vi "io.interface.vi"(7 "Caller":string, 8 "error in":errorcluster, 9 "record filename.* (disabled if empty)":string, 10 "IO Value":variant, 11 "IO Name in":string) -> (0 "error out":errorcluster, 1 "unCalibrated":u16, 2 "Value out":dbl, 3 "IoConf out":T1={"ADDR"=0, "Label"="", "Type"=enum."DI", "Mode"=enum."RIO", "Value"="", "Tags"="", "calibration"=[]} {"calibration"."Y" format="%#.3f"; "calibration"."X" format="%#.3f"; "ADDR" format="%04d"}, 4 "serialDeltaT":u32=3, 5 "DinArray out":bool[](array[boolean]))   [LabVIEW 2024]
uses:
  controls/IONode.ctl
  controls/type.address.ctl
  controls/enum.io.type.ctl
  controls/enum.io.mode.ctl
  controls/typeXyPoint.ctl
  controls/enumVarCtrlIO.ctl
  controls/cluster-com-log.ctl
  controls/enum-com-log.ctl
  <vilib>/Utility/error.llb/Clear Errors.vi
  globals/globals-engine.vi
  util.environment.vi
  util-address-parser.vi
  util-address-builder.vi
  util.DO.ToString.vi
  Polymorphics/io.command-builder.vi
  Polymorphics/io.command-builder.DO.vi
  Polymorphics/io.command-builder.AI.vi
  Polymorphics/io.command-builder.DI.vi
  io.frame.vi
  io.responseValidator.vi
  Polymorphics/io.command-parser.DI.vi
  Polymorphics/io.command-parser.AI.vi
  controls/enum.io-interface.ctl
panel:
  out "read buffer 2":string
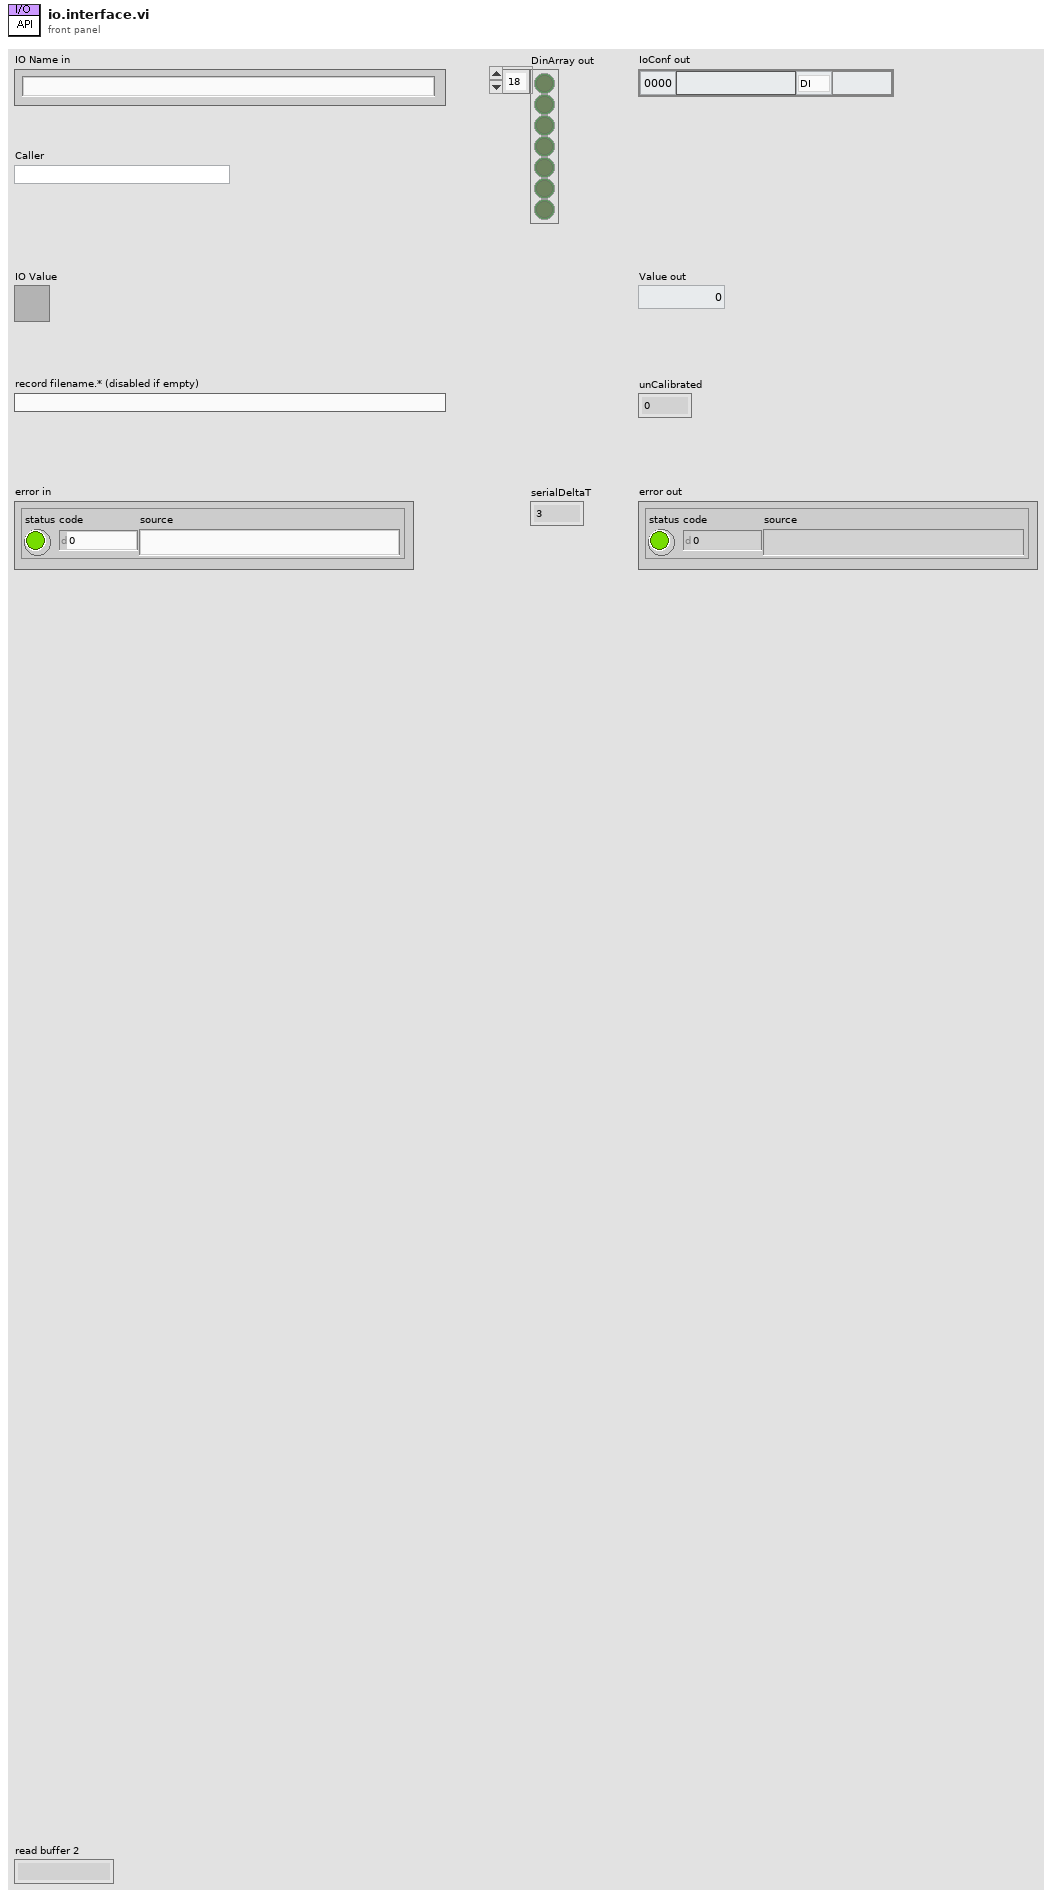
[diagram p1: front panel]
types:
  T1 = typedef "IONode.ctl" = cluster{"ADDR":T2, "Label":string, "Type":T3, "Mode":T4, "Value":string, "Tags":string, "calibration":T5[]}
  T2 = typedef "type.address.ctl" = u16
  T3 = typedef "enum.io.type.ctl" = enum16{"Type", "DI", "DO", "AI", "AO", "VL", "BUF"}
  T4 = typedef "enum.io.mode.ctl" = enum16{"Mode", "RIO", "SIM"}
  T5 = typedef "typeXyPoint.ctl" = cluster{"X":dbl, "Y":dbl}
  T6 = typedef "enum.io-interface.ctl" = enum16{"IO_VISA_WR-RD", "IO_VISA_OPEN", "IO_VISA_CLOSE", "IO_VISA_CLEAR"}
  T7 = typedef "enumVarCtrlIO.ctl" = enum16{"IO Get By Key", "IO List Configs", "IO Add By Key", "IO Modify Value By Key", "IO Modify Calib By Key", "IO Modify ADDR By Key", "IO Modify Mode By Key", "IO Modify Type By Key", "IO Modify Name By Key", "IO Remove By Key", "IO Remove All"}
  T8 = typedef "cluster-com-log.ctl" = cluster{"Caller":string, "IOnode":T1, "error":errorcluster, "dports":bool[], "AIN (calib)":dbl, "AIN (raw)":u16, "Times Stamp":timestamp, "Record File Path":path, "Visa Data":string}
  T9 = typedef "enum-com-log.ctl" = enum16{"REC.NO_OP", "REC.INIT", "REC.EXIT", "REC.SERIAL", "REC.IO", "REC.FETCH", "REC.OPEN-FILE", "REC.REOPEN-FILE"}
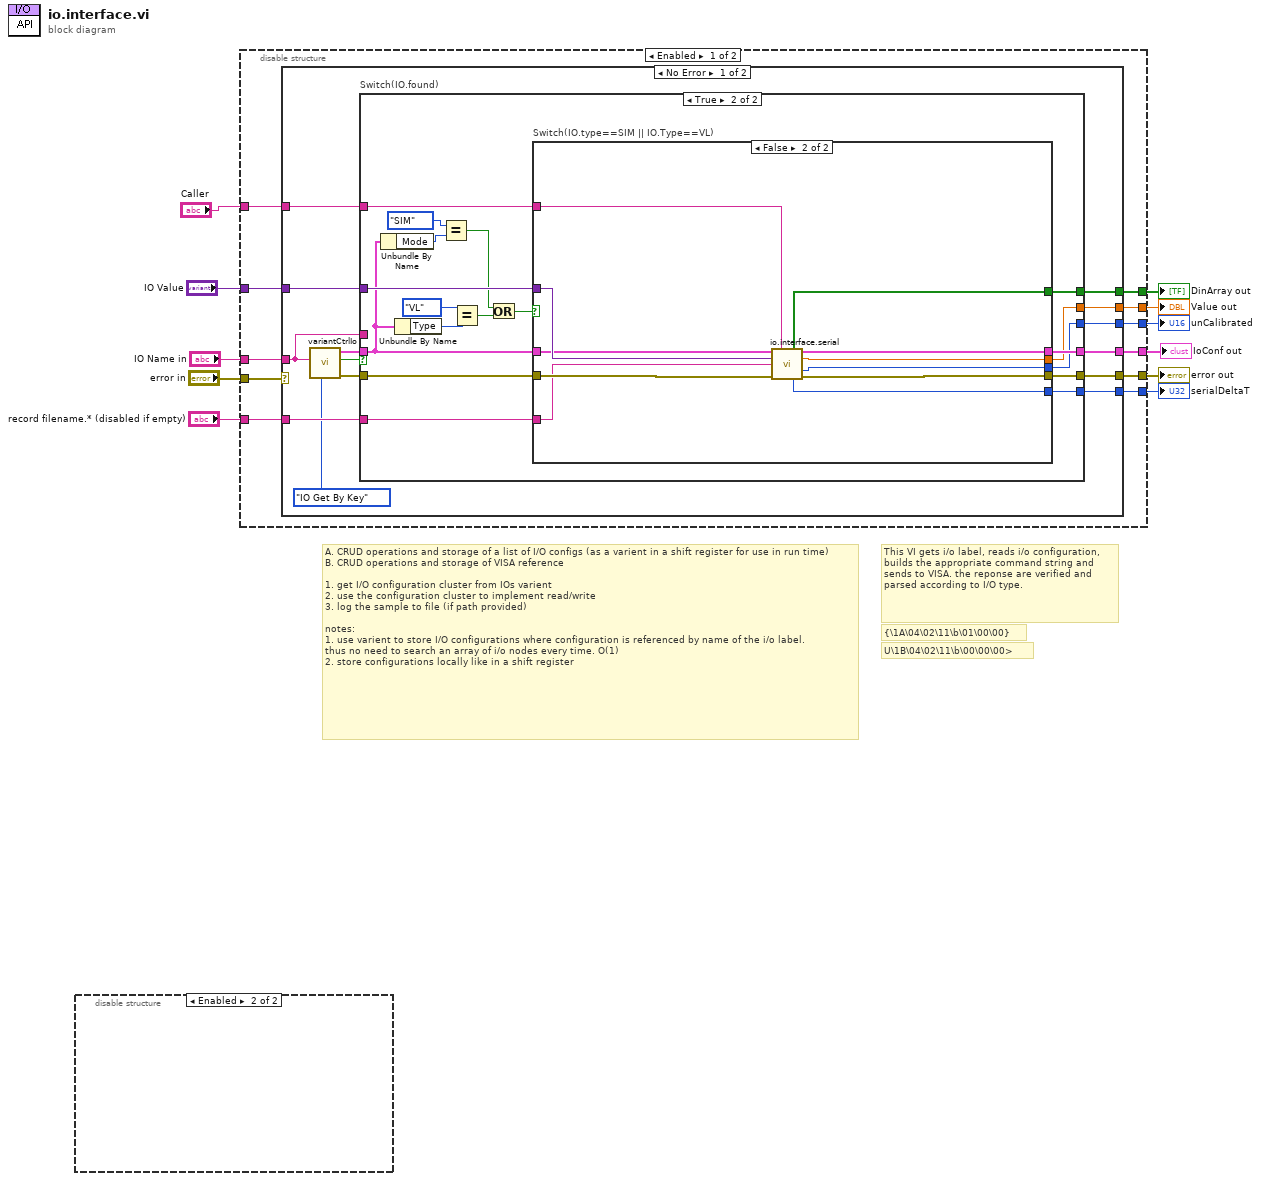
[diagram p0: block diagram]
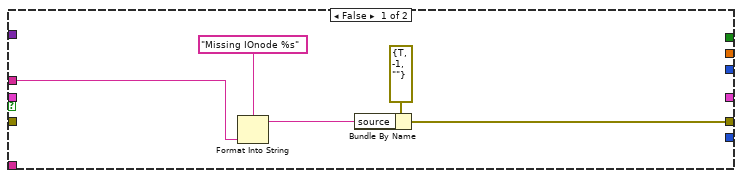
[diagram p2: hidden frame]
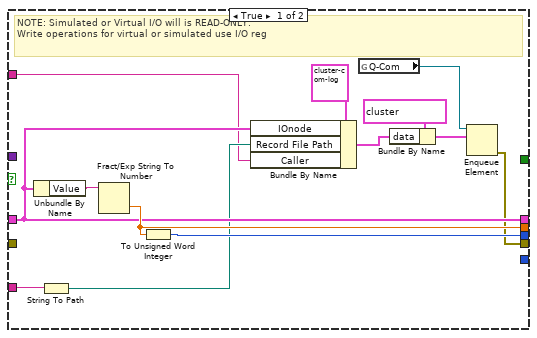
[diagram p3: hidden frame]
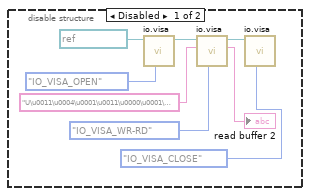
[diagram p6: hidden frame]
diagram:
  # "{\\1A\\04\\02\\11\\b\\01\\00\\00}"
  # "U\\1B\\04\\02\\11\\b\\00\\00\\00>"
  # "This VI gets i/o label, reads i/o configuration, builds the appropriate command string and sends to VISA. the reponse are verified and parsed according to I/O type."
  # "A. CRUD operations and storage of a list of I/O configs (as a varient in a shift register for use in run time)\nB. CRUD operations and storage of VISA reference\n\n1. get I/O configuration cluster from IOs varient\n2. use the configuration cluster to implement read/write \n3. log the sample to file (if path provided)\n\nnotes:\n1. use varient to store I/O configurations where configuration is referenced by name of the i/o label.\nthus no need to search an array of i/o nodes every time. O(1) \n2. store configurations locally like in a shift register"
  n1 = disable-structure shown="Enabled" {
    frame Disabled {
      n2 = call "io.visa.vi"("operation in (wr-rd)"=enum.io-interface."IO_VISA_OPEN", "VISA Refnum in"=refnum<visa-resource-name> "COM12") -> ("VISA Refnum out"=w17:refnum<visa-resource-name>)  [unwired: 6 in, 3 out]
      n3 = call "io.visa.vi"("operation in (wr-rd)"=enum.io-interface."IO_VISA_WR-RD", "write buffer"="U\u0011\u0004\u0001\u0011\u0000\u0001\u0000\u0000>" ("Command To RIO"), "VISA Refnum in"=w17) -> ("read buffer"=→"read buffer 2":string, "VISA Refnum out"=w18:refnum<visa-resource-name>)  [unwired: 5 in, 2 out]
      n4 = call "io.visa.vi"("operation in (wr-rd)"=enum.io-interface."IO_VISA_CLOSE", "VISA Refnum in"=w18) -> ()  [unwired: 6 in, 4 out]
    }
    frame Enabled {
    }
  }
  n5 = disable-structure shown="Enabled" {
    disable-tunnel: [w30 _] -> w11
    disable-tunnel: "error in" -> [w29 _]
    disable-tunnel: [w28 _] -> w9
    disable-tunnel: [w27 _] -> w8
    disable-tunnel: [w26 _] -> w2
    disable-tunnel: [w25 _] -> w7
    disable-tunnel: "record filename.* (disabled if empty)" -> [w24 _]
    disable-tunnel: "IO Value" -> [w23 _]
    disable-tunnel: "IO Name in" -> [w22 _]
    disable-tunnel: [w21 _] -> w3
    disable-tunnel: "Caller" -> [w20 _]
    frame Enabled {
      n6 = case shown="No Error" w29 {
        selector: w29 -> [_ w92]
        tunnel: [w43 w92] -> w30
        tunnel: [w44 _] -> w28
        tunnel: [w42 _] -> w27
        tunnel: [w41 _] -> w26
        tunnel: [w37 _] -> w25
        tunnel: w24 -> [w40 _]
        tunnel: w23 -> [w39 _]
        tunnel: w22 -> [w32 _]
        tunnel: [w36 _] -> w21
        tunnel: w20 -> [w31 _]
        frame No Error {
          n7 = call "variantCtrlIo.vi"("menu (Get Param)"=enumVarCtrlIO."IO Get By Key", "Key (use IOnode Label if empty )"=w32) -> ("error out"=w38:errorcluster, "found"=w33:bool, "IOnode out"=w35:T1)  [unwired: 5 in, 2 out]
          n8 = case "Switch(IO.found)" shown="True" w33 {
            tunnel: [_ w53] -> w44
            tunnel: [w45 w64] -> w43
            tunnel: [_ w52] -> w42
            tunnel: [_ w67] -> w41
            tunnel: w40 -> [_ w51]
            tunnel: w39 -> [_ w66]
            tunnel: w38 -> [_ w65]
            tunnel: [_ w63] -> w37
            tunnel: [_ w62] -> w36
            tunnel: w35 -> [_ w59]
            tunnel: w32 -> [w48 _]
            tunnel: w31 -> [_ w50]
            frame False {
              n9 = Format Into String(format string="Missing IOnode %s", w48) -> (resulting string=w47:string)  [unwired: 2 in, 1 out]
              n10 = Bundle By Name(cluster=errorcluster {"status"=TRUE, "code"=-1, "source"=""} ("input cluster"), "source"=w47) -> (w45:errorcluster)
            }
            frame True {
              n11 = Unbundle By Name(w59) -> ("Mode"=w60:T4)
              n12 = Unbundle By Name(w59) -> ("Type"=w58:T3)
              n13 = Equal?(x=enum.io.mode."SIM" ("Mode"), y=w60) -> (x = y?=w55:bool)
              n14 = Equal?(x=enum.io.type."VL", y=w58) -> (x = y?=w56:bool)
              n15 = Or(x=w55, y=w56) -> (x .or. y?=w54:bool)
              n16 = case "Switch(IO.type==SIM || IO.Type==VL)" shown="False" w54 {
                tunnel: w66 -> [_ w91]
                tunnel: [w79 w85] -> w53
                tunnel: [w71 w90] -> w64
                tunnel: w65 -> [_ w89]
                tunnel: [_ w84] -> w67
                tunnel: w59 -> [w73 w88]
                tunnel: [w78 w87] -> w52
                tunnel: [_ w86] -> w62
                tunnel: [w73 w83] -> w63
                tunnel: w51 -> [w70 w82]
                tunnel: w50 -> [w68 w81]
                frame True {
                  # "NOTE: Simulated or Virtual I/O will is READ-ONLY. \nWrite operations for virtual or simulated use I/O reg"
                  n17 = Unbundle By Name(w73) -> ("Value"=w80:string)
                  n18 = String To Path(string=w70) -> (path=w69:path)
                  n19 = Fract/Exp String To Number(string=w80) -> (number=w79:dbl)  [unwired: 3 in, 1 out]
                  n20 = To Unsigned Word Integer(number=w79) -> (unsigned 16bit integer=w78:u16)
                  n21 = Bundle By Name(cluster=T8 {"Caller"="", "IOnode"={"ADDR"=0, "Label"="Name", "Type"=enum."DI", "Mode"=enum."RIO", "Value"="Value", "Tags"="Tags", "calibration"=[]}, "error"={"status"=FALSE, "code"=0, "source"=""}, "dports"=[], "AIN (calib)"=0.0, "AIN (raw)"=0, "Times Stamp"=timestamp(0 s since 1904-01-01), "Record File Path"=path "", "Visa Data"=""} ("input cluster"), "IOnode"=w73, "Record File Path"=w69, "Caller"=w68) -> (w72:T8)
                  n22 = global read "globals-engine.vi" "Q-Com"() -> (w76:refnum<queue>)
                  n23 = Bundle By Name(cluster=cluster{"data":variant, "Enum":T9} {"data"=variant, "Enum"=enum."REC.IO"} ("procQ"), "data"=w72) -> (w77:cluster{"data":variant, "Enum":T9})
                  n24 = Enqueue Element(queue=w76, element=w77) -> (error out=w71:errorcluster)  [unwired: 2 in, 2 out]
                }
                frame False {
                  n25 = call "io.interface.serial.vi"("IoConf in"=w88, "Caller"=w81, "Output State"=w91, "record filename.* (disabled if empty)"=w82, "error in (no error)"=w89) -> ("DI"=w86:bool[], "IoConf out"=w83:T1, "IN (calib)"=w85:dbl, "IN (uncalib)"=w87:u16, "Operation Time ms"=w84:u32, "error out"=w90:errorcluster)  [unwired: 5 in]
                }
              }
            }
          }
        }
        frame Error {
        }
      }
    }
    frame Disabled {
    }
  }
  "error out" <- w11
  "Value out" <- w9
  "unCalibrated" <- w8
  "serialDeltaT" <- w2
  "DinArray out" <- w3
  "IoConf out" <- w7
